vi "MoveToTarget.vi"(8 "error in":errorcluster, 9 "DecFactor":fxp<+,16,16>=100.0, 10 "CursLoc":cluster{"X":dbl, "Y":dbl}, 11 "Target in":cluster{"x":dbl, "y":dbl}) -> (0 "error out":errorcluster, 2 "target -1":cluster{"x":dbl, "y":dbl}, 3 "Target out":cluster{"x":dbl, "y":dbl})   [LabVIEW 2016]
uses:
  controls/Enum.ctl
  <vilib>/Utility/error.llb/Error Cluster From Error Code.vi
  <vilib>/rvi/errors/niLvFpgaAdjustHostInterfaceError.vi
  <vilib>/rvi/interface/nirviReadWriteControl/nirviReadWriteControl.xnode
  controls/FPGAVIreferenceTypeDefScanEngine.ctl
  FPGA Bitfiles/qnmController797_usbRIO_controllerFPGAmu.lvbitx
  NiFpgaLv.dll
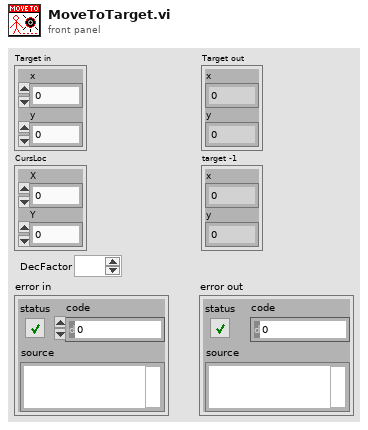
[diagram p1: front panel]
types:
  T1 = typedef "Enum.ctl" = enum16{"Init", "Read", "Write"}
  T2 = cluster{"calibName":string[], "calibParameters":cluster{"Sensitivity":cluster{"Sens X":dbl, "Sens Y":dbl, "Sens Z":dbl}, "Range":cluster{"Range X":dbl, "Range Y":dbl, "Range Z":dbl}, "HV gain":cluster{"HV gain X":dbl, "HV gain Y":dbl, "HV gain Z":dbl}}[], "calibIndex":i32}
  T3 = cluster{"Sensitivity":cluster{"Sens X":dbl, "Sens Y":dbl, "Sens Z":dbl}, "Range":cluster{"Range X":dbl, "Range Y":dbl, "Range Z":dbl}, "HV gain":cluster{"HV gain X":dbl, "HV gain Y":dbl, "HV gain Z":dbl}}[]
  T4 = cluster{"Width":dbl, "Height":dbl, "X Offset":dbl, "Y Offset":dbl, "Angle":dbl, "Pixels/Line":u16, "Lines":u16, "Time/Line":dbl, "Scan Rate":dbl}
  T5 = cluster{"Sensitivity":cluster{"Sens X":dbl, "Sens Y":dbl, "Sens Z":dbl}, "Range":cluster{"Range X":dbl, "Range Y":dbl, "Range Z":dbl}, "HV gain":cluster{"HV gain X":dbl, "HV gain Y":dbl, "HV gain Z":dbl}}
  T6 = typedef "FPGAVIreferenceTypeDefScanEngine.ctl" = refnum<k20>
  T7 = cluster{"moveToDecFactor":u16, "moveToWaveSize":u16, "se.mot.p.invDec":fxp<+,16,0>}
  T8 = cluster{"se.p.enable":bool, "se.p.singleDirection":bool, "se.p.haltScan":bool, "se.mot.p.start":bool}
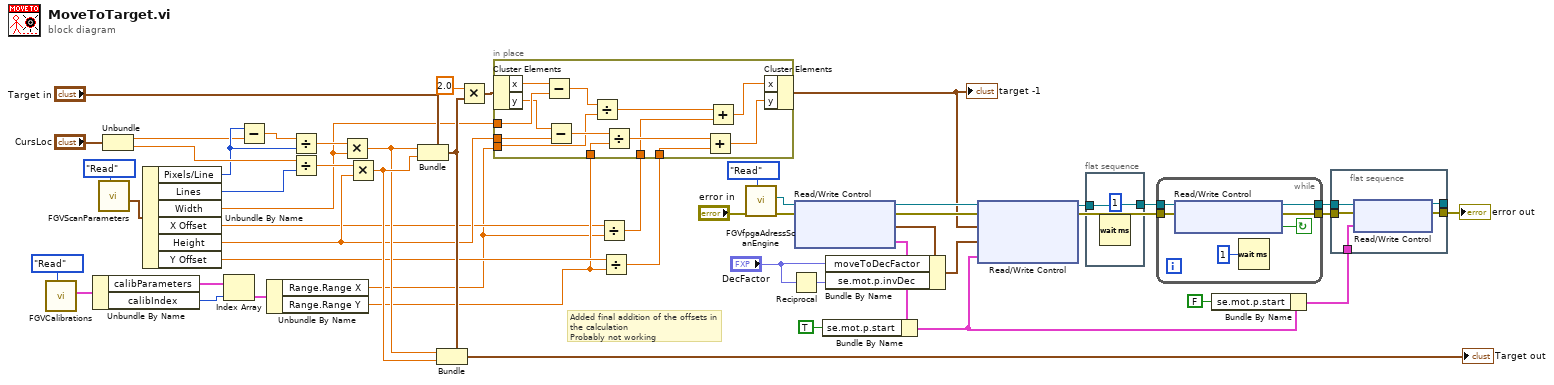
[diagram p0: block diagram]
diagram:
  # "Added final addition of the offsets in the calculation\nProbably not working"
  n1 = call "FGVCalibrations.vi"("Enum"=Enum."Read") -> ("calibOut"=w24:T2)  [unwired: 9 in, 1 out]
  n2 = Unbundle By Name(w24) -> ("calibParameters"=w25:T3, "calibIndex"=w26:i32)
  n3 = call "FGVScanParameters.vi"("Enum"=Enum."Read") -> ("Scan Parameters Out"=w29:T4)  [unwired: 9 in, 1 out]
  n4 = Unbundle("CursLoc") -> ("X"=w10:dbl, "Y"=w22:dbl)
  n5 = Unbundle By Name(w29) -> ("Pixels/Line"=w11:u16, "Lines"=w21:u16, "Width"=w12:dbl, "X Offset"=w5:dbl, "Height"=w13:dbl, "Y Offset"=w7:dbl)
  n6 = Index Array(array=w25, index=w26) -> (element=w27:T5)
  n7 = Subtract(x=w11, y=w10) -> (x-y=w9:dbl)
  n8 = Unbundle By Name(w27) -> ("Range.Range X"=w4:dbl, "Range.Range Y"=w6:dbl)
  n9 = Divide(x=w9, y=w11) -> (x/y=w18:dbl)
  n10 = Divide(x=w22, y=w21) -> (x/y=w19:dbl)
  n11 = Multiply(x=w18, y=w12) -> (x*y=w14:dbl)
  n12 = Multiply(x=w19, y=w13) -> (x*y=w15:dbl)
  n13 = Bundle(cluster="Target in", "x"=w14, "y"=w15) -> (w17:cluster{"x":dbl, "y":dbl})
  n14 = Bundle(cluster=w17, "x"=w14, "y"=w15) -> (→"Target out":cluster{"x":dbl, "y":dbl})
  n15 = Multiply(x=2.0, y=w17) -> (x*y=w2:cluster{"x":dbl, "y":dbl})
  n16 = Divide(x=w5, y=w4) -> (x/y=w3:dbl)
  n17 = Divide(x=w7, y=w6) -> (x/y=w8:dbl)
  n18 = in-place {
    in-place-border: w13 -> [w64]
    in-place-border: w12 -> [w63]
    in-place-border: w8 -> [w62]
    in-place-border: w6 -> [w60]
    in-place-border: w4 -> [w58]
    in-place-border: w3 -> [w57]
    n19 = in-place-cluster #1(w2) -> ("x"=w56:dbl, "y"=w55:dbl)
    n20 = Subtract(x=w56, y=w63) -> (x-y=w66:dbl)
    n21 = Subtract(x=w55, y=w64) -> (x-y=w65:dbl)
    n22 = Divide(x=w66, y=w58) -> (x/y=w59:dbl)
    n23 = Divide(x=w65, y=w60) -> (x/y=w61:dbl)
    n24 = Add(x=w61, y=w62) -> (x+y=w53:dbl)
    n25 = Add(x=w59, y=w57) -> (x+y=w54:dbl)
    n26 = in-place-cluster #1("x"=w54, "y"=w53) -> (w1:cluster{"x":dbl, "y":dbl})
  }
  "target -1" <- w1
  n27 = call "FGVfpgaAdressScanEngine.vi"("Enum"=Enum."Read", "error in"="error in") -> ("error out"=w32:errorcluster, "FPGA.SEout"=w33:T6)  [unwired: 5 in, 3 out]
  n28 = Reciprocal(x="DecFactor") -> (1/x=w46:fxp<+,17,1>)
  n29 = xnode "Read/Write Control"("FPGA VI Reference In"=w33, "error in"=w32) -> ("FPGA VI Reference Out"=w49:T6, "error out"=w48:errorcluster, "se.mot.p.clocks"=w35:T7, "se.p.modes"=w47:T8)
  n30 = Bundle By Name(cluster=w47, "se.mot.p.start"=TRUE) -> (w40:T8)
  n31 = Bundle By Name(cluster=w35, "moveToDecFactor"="DecFactor", "se.mot.p.invDec"=w46) -> (w44:T7)
  n32 = xnode "Read/Write Control"("FPGA VI Reference In"=w49, "error in"=w48, "se.mot.p.target"=w1, "se.mot.p.clocks"=w44, "se.p.modes"=w40) -> ("FPGA VI Reference Out"=w37:T6, "error out"=w31:errorcluster)
  n33 = flat-sequence {
    tunnel: [w68] -> w38
    tunnel: w37 -> [w68]
    frame #0 {
      n34 = Wait (ms)(milliseconds to wait=u32 1) -> ()  [unwired: 1 out]
    }
  }
  n35 = while {
    tunnel: w38 -> [w74]
    tunnel: w31 -> [w73]
    tunnel: [w72] -> w42
    tunnel: [w70] -> w41
    stop <- w71 continue-if-true
    n36 = xnode "Read/Write Control"("FPGA VI Reference In"=w74, "error in"=w73) -> ("FPGA VI Reference Out"=w72:T6, "error out"=w70:errorcluster, "se.mot.s.running"=w71:bool)
    n37 = Wait (ms)(milliseconds to wait=u32 1) -> ()  [unwired: 1 out]
  }
  n38 = Bundle By Name(cluster=w40, "se.mot.p.start"=FALSE) -> (w43:T8)
  n39 = flat-sequence {
    tunnel: w41 -> [w77]
    tunnel: w42 -> [w79]
    tunnel: [w78] -> _
    tunnel: w43 -> [w76]
    tunnel: [w75] -> w51
    frame #0 {
      n40 = xnode "Read/Write Control"("FPGA VI Reference In"=w79, "error in"=w77, "se.p.modes"=w76) -> ("FPGA VI Reference Out"=w78:T6, "error out"=w75:errorcluster)
    }
  }
  "error out" <- w51
